vi "PasswordReset.vi"(7 "NEW PASSWORD":string, 8 "error in":errorcluster, 9 "User Cred":T1, 10 "Authenticated Data":string[][](array[string]), 11 "OLD PASSWORD":string) -> (0 "error out":errorcluster)   [LabVIEW 2022 SP3]
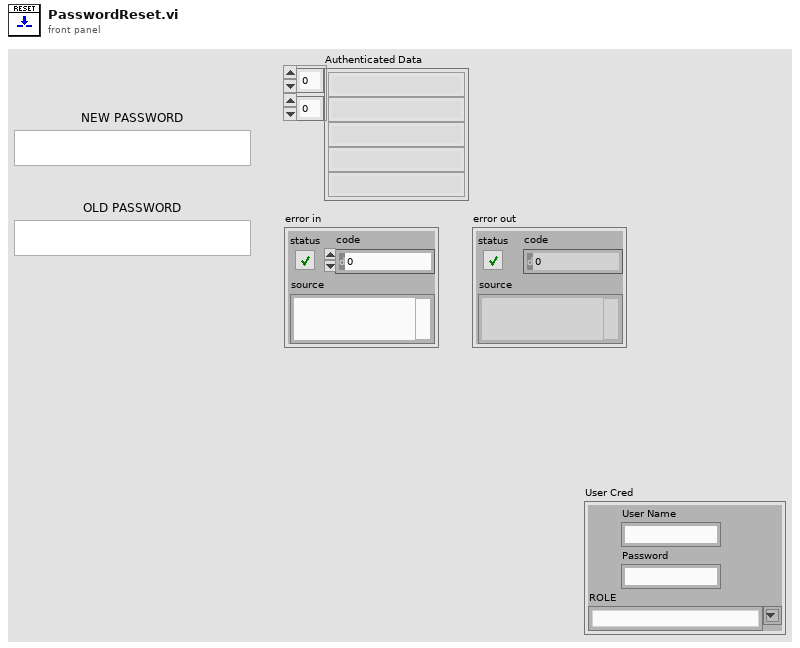
[diagram p1: front panel]
types:
  T1 = cluster{"User Name":string, "Password":string, "ROLE":string}
  T2 = enum16{"Initialize", "Verify User", "Change Password", "Wrong Cred", "Exit"}
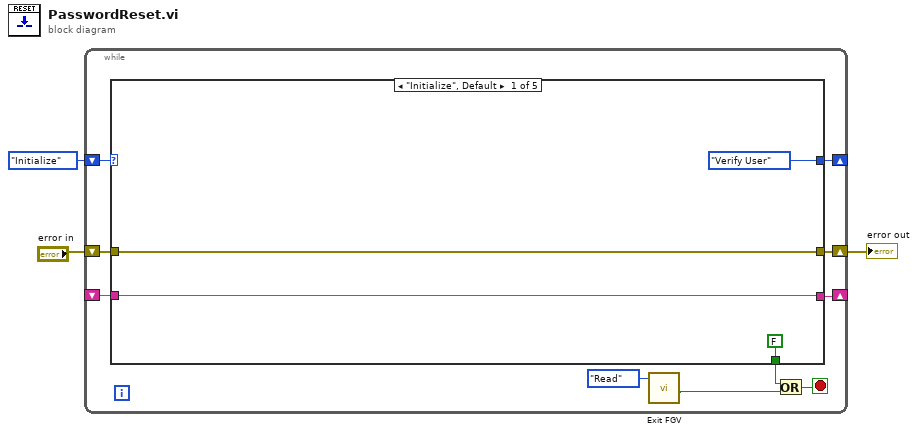
[diagram p0: block diagram]
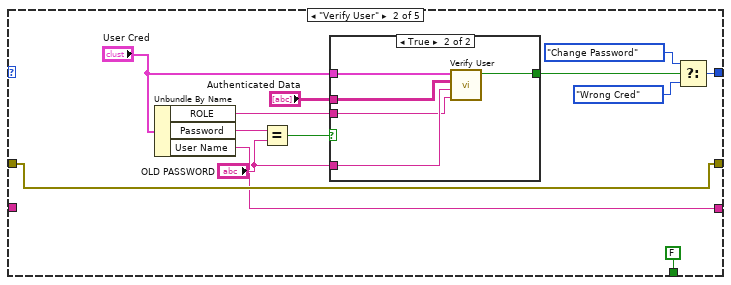
[diagram p2: hidden frame]
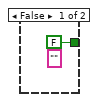
[diagram p3: hidden frame]
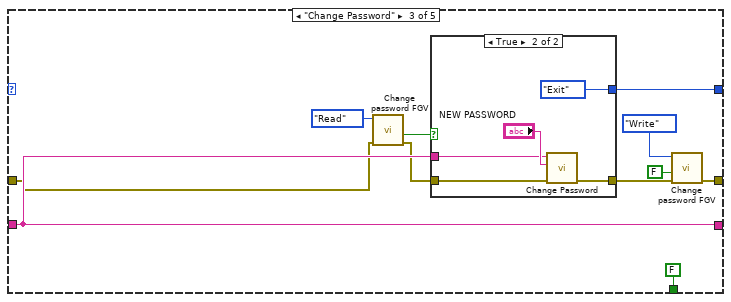
[diagram p4: hidden frame]
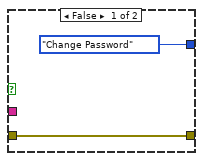
[diagram p5: hidden frame]
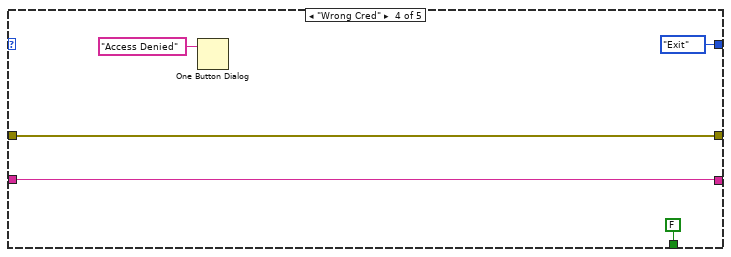
[diagram p6: hidden frame]
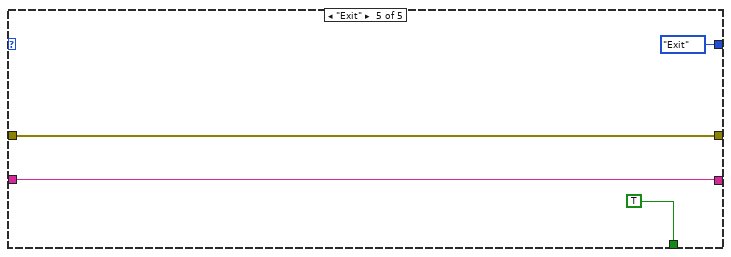
[diagram p7: hidden frame]
diagram:
  n1 = while {
    shift-right: [w12] -> _
    shift-left: T2."Initialize" -> [w13]
    shift-right: [w9] -> w1
    shift-left: "error in" -> [w8]
    shift-right: [w7] -> _
    shift-left: _ -> [w6]
    stop <- w11 stop-if-true
    n2 = case shown="\"Initialize\", Default" w13 {
      tunnel: [T2."Verify User" w28 w47 T2."Exit" ("f") T2."Exit" ("f")] -> w12
      tunnel: [FALSE ("x") FALSE ("x") FALSE ("x") FALSE ("x") TRUE ("x")] -> w10
      tunnel: [w15 w22 w37 w56 w61] -> w9
      tunnel: w8 -> [w15 w22 w42 w56 w61]
      tunnel: [w14 w18 w45 w55 w60] -> w7
      tunnel: w6 -> [w14 _ w45 w55 w60]
      frame "Initialize", Default {
      }
      frame "Verify User" {
        n3 = Unbundle By Name("User Cred") -> ("ROLE"=w19:string, "Password"=w25:string, "User Name"=w18:string)
        n4 = Equal?(x=w25, y="OLD PASSWORD") -> (x = y?=w24:bool)
        n5 = case shown="True" w24 {
          tunnel: [FALSE ("Boolean") w33] -> w26
          tunnel: "User Cred" -> [_ w36]
          tunnel: "Authenticated Data" -> [_ w35]
          tunnel: "OLD PASSWORD" -> [_ w34]
          tunnel: w19 -> [_ w32]
          frame False {
            (unwired) "" ("OLD PASSWORD out")
          }
          frame True {
            n6 = call "Verify User.vi"("ROLE"=w32, "OLD PASSWORD in"=w34, "Authenticated Data"=w35, "User Cred"=w36) -> ("Password True?"=w33:bool)  [unwired: 5 in, 2 out]
          }
        }
        n7 = Select(t=T2."Change Password", s=w26, f=T2."Wrong Cred") -> (s? t:f=w28:T2)
      }
      frame "Change Password" {
        n8 = call "Change password FGV.vi"("error in"=w42, "Enum"=enum16{"Read", "Write"}."Read") -> ("error Out"=w41:errorcluster, "Change Password Out"=w43:bool)  [unwired: 8 in]
        n9 = case shown="True" w43 {
          tunnel: [T2."Change Password" ("f") T2."Exit" ("f")] -> w47
          tunnel: w41 -> [w48 w52]
          tunnel: [w48 w50] -> w38
          tunnel: w45 -> [_ w51]
          frame False {
          }
          frame True {
            n10 = call "Change Password.vi"("error in"=w52, "New Password"="NEW PASSWORD", "User Name"=w51) -> ("error out"=w50:errorcluster)  [unwired: 8 in]
          }
        }
        n11 = call "Change password FGV.vi"("error in"=w38, "Change Password in"=FALSE, "Enum"=enum16{"Read", "Write"}."Write") -> ("error Out"=w37:errorcluster)  [unwired: 7 in, 1 out]
      }
      frame "Wrong Cred" {
        n12 = One Button Dialog(message="Access Denied") -> ()  [unwired: 1 in, 1 out]
      }
      frame "Exit" {
      }
    }
    n13 = call "Exit FGV.vi"("Enum"=enum16{"Read", "Write"}."Read") -> ("Exit Out"=w4:bool)  [unwired: 10 in]
    n14 = Or(x=w10, y=w4) -> (x .or. y?=w11:bool)
  }
  "error out" <- w1
